vi "Trigger_measurement.vi"() -> ()   [LabVIEW 2024]
doc: "This example performs writes and reads on a serial port, as directed by the user. You can press the Write and Read buttons, and change the Read Count, while the example is running.\n\nThe parameters set for the serial port must match the parameters of the connected instrument or device. In this example, the Read Count parameter specifies the number of bytes that the serial port reads. If there were more bytes at the port than the specified number, those bytes would not be read. If there were less bytes at the port than the specified number, you would receive a timeout error.\n\nThis example expands upon the flow control options for XON and XOFF, allowing the user to choose those control characters. Also, the user can enable or disable a termination character. Some devices require a termination character in order to identify the end of command strings. Some devices send a termination character to signify the end of data to be read. This example shows how you can end the Read operation once a termination character is detected in the buffer and/or append a termination character at the end of the Write data."
uses:
  support/Serial - ASCII Characters.ctl
  support/Serial - XON-XOFF Characters.ctl
  support/Serial - Settings.ctl
  <vilib>/Instr/_visa.llb/VISA Configure Serial Port (Instr).vi
panel:
  in  "Measure?":bool
  out "Response":string
  # "Overview: Demonstrates the use of the VISA functions to write commands to and read responses from a serial instrument continuously in a loop.\nRequirements: NI-VISA Driver\nInstructions:\n1. Run the VI.\n2. Specify a Command and click the Write button.\n3. Read a Response by clicking the Read button.\n4. Click Stop to stop the VI."
  # "0xA is equivalent to a '\\n' character, which is a line feed."
  # "Multi-Commands can be given in one command if seperated by semicolons"
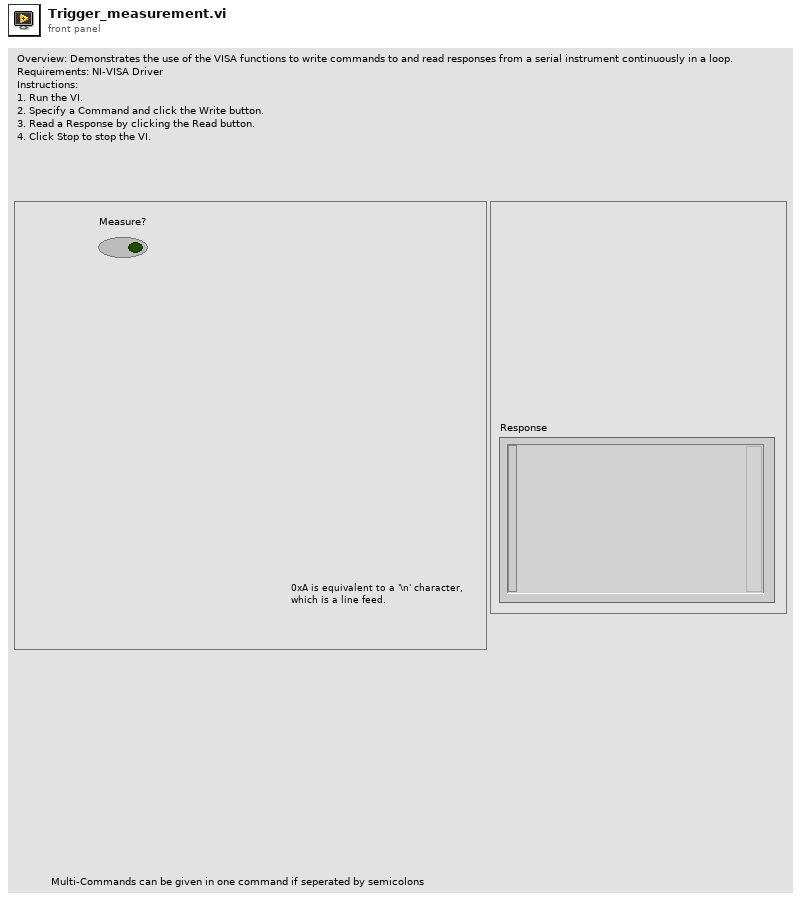
[diagram p1: front panel]
types:
  T1 = typedef "Serial - Settings.ctl" = cluster{"baud rate":u32, "data bits":u16, "parity":enum16{"None", "Odd", "Even", "Mark", "Space"}, "stop bits":u16, "flow control":u16}
  T2 = typedef "Serial - XON-XOFF Characters.ctl" = cluster{"XON":T3, "XOFF":T3}
  T3 = typedef "Serial - ASCII Characters.ctl" = enum16{"NUL", "SOH", "STX", "ETX", "EOT", "ENQ", "ACK", "BEL", "BS", "HT", "LF", "VT", "FF", "CR", "SO", "SI", "DLE", "DC1", "DC2", "DC3", "DC4", "NAK", "SYN", "ETB", "CAN", "EM", "SUB", "ESC", "FS", "GS", "RS", "US", "SP", "!", "\"", "#", "$", "%", "&", "'", "(", ")", "*", "+", ",", "- (-)", ".", "/", "0", "1", "2", "3", "4", "5", "6", "7", "8", "9", ":", ";", "<", "=", ">", "?", "@", "A", "B", "C", "D", "E", "F", "G", "H", "I", "J", "K", "L", "M", "N", "O", "P", "Q", "R", "S", "T", "U", "V", "W", "X", "Y", "Z", "[", "\\", "]", "^", "_", "`", "a", "b", "c", "d", "e", "f", "g", "h", "i", "j", "k", "l", "m", "n", "o", "p", "q", "r", "s", "t", "u", "v", "w", "x", "y", "z", "{", "|", "}", "~"}
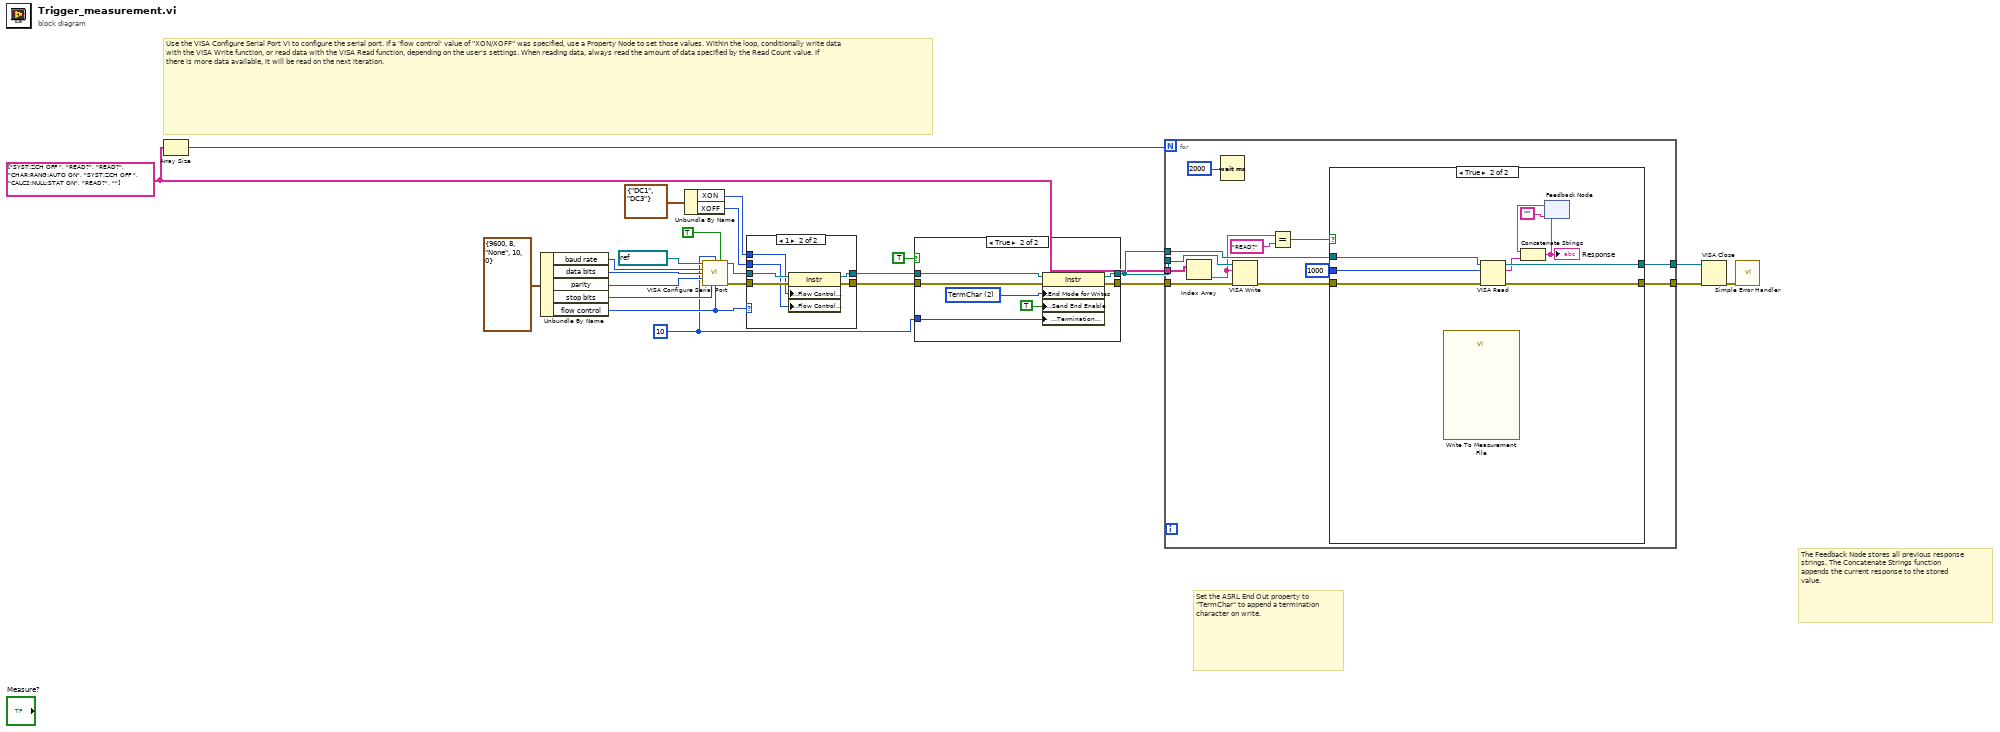
[diagram p0: block diagram]
diagram:
  w1 = string[] ["SYST:ZCH OFF ", "READ?", "READ?", "CHAR:RANG:AUTO ON", "SYST:ZCH OFF ", "CALC2:NULL:STAT ON", "READ?", ""] ("Commands")
  w3 = u8 10 ("Termination Character")
  # "The Feedback Node stores all previous response strings. The Concatenate Strings function appends the current response to the stored value."
  # "Set the ASRL End Out property to \"TermChar\" to append a termination character on write."
  # "Use the VISA Configure Serial Port VI to configure the serial port. If a 'flow control' value of \"XON/XOFF\" was specified, use a Property Node to set those values. Within the loop, conditionally write data with the VISA Write function, or read data with the VISA Read function, depending on the user's settings. When reading data, always read the amount of data specified by the Read Count value. If there is more data available, it will be read on the next iteration."
  n1 = Array Size(array=w1) -> (size(s)=w2:i32)
  n2 = Unbundle By Name(T1 {"baud rate"=9600, "data bits"=8, "parity"=enum."None", "stop bits"=10, "flow control"=0} ("Serial Settings")) -> ("baud rate"=w17:u32, "data bits"=w18:u16, "parity"=w19:enum16{"None", "Odd", "Even", "Mark", "Space"}, "stop bits"=w20:u16, "flow control"=w11:u16)
  n3 = Unbundle By Name(T2 {"XON"=enum."DC1", "XOFF"=enum."DC3"} ("XON/XOFF Characters")) -> ("XON"=w10:T3, "XOFF"=w9:T3)
  n4 = call-poly "VISA Configure Serial Port"("VISA resource name"=refnum<visa-resource-name> "COM1", "termination char\n(0xA = '\\n' = LF)"=w3, "Enable Termination\nChar (T)"=TRUE ("End Read on Termination Character?"), "baud rate (9600)"=w17, "data bits (8)"=w18, "parity (0:none)"=w19, "stop bits (10: 1 bit)"=w20, "flow control (0:none)"=w11) -> ("VISA resource name out"=w21:refnum<visa-resource-name>, "error out"=w22:errorcluster)  [unwired: 2 in, 4 out]
  n5 = case shown="1" w11 {
    tunnel: [w25 w32] -> w8
    tunnel: [w26 w31] -> w6
    tunnel: w22 -> [w25 w30]
    tunnel: w21 -> [w26 w29]
    tunnel: w10 -> [_ w28]
    tunnel: w9 -> [_ w27]
    frame Default {
    }
    frame 1 {
      n6 = property class="Instr"(reference=w29, error in=w30, "Serial Settings:Flow Control XON Character"=w28, "Serial Settings:Flow Control XOFF Character"=w27) -> (reference out=w31:refnum<visa-resource-name>, error out=w32:errorcluster)
    }
  }
  n7 = case shown="True" TRUE ("End Write on Termination Character?") {
    tunnel: w6 -> [w33 w41]
    tunnel: w8 -> [w34 w40]
    tunnel: [w33 w39] -> w5
    tunnel: [w34 w38] -> w7
    tunnel: w3 -> [_ w36]
    frame False {
    }
    frame True {
      w37 = u16 2 items=["None", "LastBit", "TermChar", "Break"] ("Serial Settings:Serial End Mode for Writes")
      n8 = property class="Instr"(reference=w41, error in=w40, "Serial Settings:End Mode for Writes"=w37, "Message Based Settings:Send End Enable"=TRUE, "Message Based Settings:Termination Character"=w36) -> (reference out=w39:refnum<visa-resource-name>, error out=w38:errorcluster)
    }
  }
  n9 = for {
    N: w2 -> [_]
    tunnel: w1 -> [w53]
    tunnel: w5 -> [w52]
    tunnel: w7 -> [w50]
    tunnel: [w45] -> w12
    tunnel: [w46] -> w13
    tunnel: w5 -> [w47]
    n10 = Index Array(array=w53) -> (element=w43:string)  [unwired: 1 in]
    n11 = Wait (ms)(milliseconds to wait=u32 2000) -> ()  [unwired: 1 out]
    n12 = VISA Write(VISA resource name=w52, write buffer=w43, error in (no error)=w50) -> (error out=w49:errorcluster)  [unwired: 2 out]
    n13 = Equal?(x=w43, y="READ?") -> (x = y?=w44:bool)
    n14 = case shown="True" w44 {
      tunnel: w49 -> [w54 w64]
      tunnel: u32 1000 ("Read Count") -> [_ w63]
      tunnel: w47 -> [w55 w62]
      tunnel: [w54 w61] -> w46
      tunnel: [w55 w60] -> w45
      frame False {
      }
      frame True {
        n15 = call "Write To Measurement File"() -> ()  [unwired: 17 in, 3 out]
        n16 = VISA Read(VISA resource name=w62, byte count=w63, error in (no error)=w64) -> (VISA resource name out=w60:refnum<visa-resource-name>, read buffer=w57:string, error out=w61:errorcluster)  [unwired: 1 out]
        n17 = feedback #1("") -> (w59:string)
        n18 = Concatenate Strings(w59, w57) -> (w56:string)
        "Response" <- w56
        n19 = feedback-in #1(w56) -> ()
      }
    }
  }
  n20 = VISA Close(VISA resource name=w12, error in (no error)=w13) -> (error out=w14:errorcluster)
  n21 = call <vilib>:"Simple Error Handler.vi"("error in (no error)"=w14) -> ()  [unwired: 1 in, 8 out]
